vi "MEASURE_hysteresis_multiple_SHG gate_pmt-final - Set voltage.vi"() -> ()   [LabVIEW 2020]
uses:
  <vilib>/DAQmx/read.llb/DAQmx Read.vi
  <vilib>/DAQmx/read.llb/DAQmx Read (Counter U32 1Chan 1Samp).vi
  <vilib>/Analysis/baseanly.llb/Mean (DBL).vi
  <vilib>/DAQmx/create/channels.llb/DAQmx Create Channel (CI-Count Edges).vi
  Program Files/National Instruments/LabVIEW 2019/instr.lib/Keithley 24XX/Public/Data/Read (Multiple Points).vi
  <vilib>/DAQmx/miscellaneous.llb/DAQmx Fill In Error Info.vi
  <vilib>/Utility/file.llb/Write To Spreadsheet File (DBL).vi
  Program Files/National Instruments/LabVIEW 2019/instr.lib/Stanford Research 830/Stanford Research 830.lvlib
  <resource>/objmgr/daqmx.rc
  Program Files/National Instruments/LabVIEW 2019/instr.lib/Keithley 24XX/Keithley 24XX.lvlib
  <vilib>/Analysis/NI_AALBase.lvlib
panel:
  in  "Set voltage (T)":bool=TRUE
  in  "back Vg final Value":dbl=6.0
  in  "Gate sequence":dbl
  out "while loop":dbl
  in  "bottom gate-off set":dbl=-5.0
  in  "0ff set{T}/no off set[F]":bool
  out "XY Graph 4":cluster{dbl[], dbl[]}(graph)
  out "XY Graph 3":cluster{dbl[], dbl[]}(graph)
  out "back gate leaking":dbl=2.469318360898143e-10
  out "top gate voltage":dbl format="%#_13g"
  in  "Compliance  Level (1uA)":dbl=1.9999999995789155e-07
  in  "Source Mode  (0: Voltage)":u16(ring) items=["Voltage", "Current"]
  in  "Serial Configuration":T1={"Baud Rate"=9600, "Parity"=0, "Data Bits"=8, "Stop Bits"=10, "Flow Control"=0} {"Flow Control" items=["None", "XON/XOFF", "RTS/CTS", "XON/XOFF & RTS/CTS", "DTR/DSR", "XON/XOFF & DTR/DSR"]; "Stop Bits" items=["1.0"=10, "1.5"=15, "2.0"=20]; "Data Bits" items=["7"=7, "8"=8]; "Parity" items=["None", "Odd", "Even", "Mark", "Space"]; "Baud Rate" items=["300"=300, "600"=600, "1200"=1200, "2400"=2400, "4800"=4800, "9600"=9600, "19200"=19200]}
  in  "back gate address":refnum<visa-resource-name>="GPIB0::25::INSTR"
  in  "top gate thickness":dbl=10.0
  in  "back gate thickness":dbl=30.0
  in  "pure field (T)/pure doping (F)":bool
  in  "Clear Plot 2":bool
  out "XY Graph 2":cluster{dbl[], dbl[]}(graph)
  in  "accumulation":i32=80
  out "Waveform Chart 3":dbl[](graph)=[376.0, 339.0, 337.0, 347.0, 368.0, 343.0, 313.0, 342.0, 356.0, 353.0, 315.0, 360.0, 375.0, 301.0, 363.0, 324.0, 334.0, 324.0, 318.0, 329.0, 312.0, 341.0, 352.0, 336.0, 351.0, 312.0, 361.0, 339.0, 352.0, 315.0, 360.0, 366.0, 324.0, 343.0, 343.0, 330.0, 340.0, 327.0, 393.0, 330.0, 335.0, 353.0, 360.0, 347.0, 337.0, 336.0, 312.0, 331.0, 326.0, 350.0, 344.0, 328.0, 357.0, 355.0, 356.0, 331.0, 328.0, 340.0, 355.0, 387.0, 371.0, 360.0, 331.0, 339.0, 344.0, 367.0, 343.0, 360.0, 360.0, 370.0, 335.0, 366.0, 323.0, 378.0, 373.0, 358.0]
  out "Numeric":dbl=344.60526315789474
  in  "Counter Channel":tag="/Dev1/PFI0"
  in  "error in":errorcluster
  out "loop run":i32=2
  in  "loop #":i32=2
  in  "Save data or not":bool=TRUE
  in  "path (folder + filename)":string="C:\\Users\\User\\Data\\Jason\\03282019\\ pure_bottom_high_6v_rato3 with light2"
  in  "Clear Plot":bool
  out "LOCKIN Measurement":dbl=0.9110010000000001
  in  "Parameter (1: X)":u16(ring)=1 items=["X"=1, "Y"=2, "R"=3, "Theta"=4, "Channel 1"=5, "Channel 2"=6, "Aux In 1"=7, "Aux In 2"=8, "Aux In 3"=9, "Aux In 4"=10]
  out "back gate voltage":dbl format="%#_13g"
  out "top gate leaking":string="-9.306248E-12\n"
  in  "GATE STEP(mv)":i32=450
  in  "GATE Low Value (default 0)":dbl
  in  "GATE High Value":dbl=18.0
  in  "Function (0: Volts) 2":u16(ring) items=["Volts", "Current", "Resistance"]
  in  "Source Compaliance":dbl=1.000000000000001e-07
  in  "topgate address":refnum<visa-resource-name>="GPIB0::18::INSTR"
  in  "SD stabilization(S) 2":dbl=0.1 format="%#_13g"
  in  "Sine Output Amplitude (1 V) 2":dbl=0.05
  in  "GATE / SD stablization 3":dbl=0.1 format="%#_13g"
  in  "frequency":dbl=50.0 format="%#_13g"
  in  "Input Connection (0: Single-Ended Voltage)":u16(ring) items=["Single-Ended Voltage", "Differential Voltage", "1 MOhm Current Gain", "100 MOhm Current Gain"]
  in  "LOCKIN address":refnum<visa-resource-name>="GPIB0::8::INSTR"
  # "Gate2400(top) Setting"
  # "Lock-in"
  # "Gate2400(back) Setting"
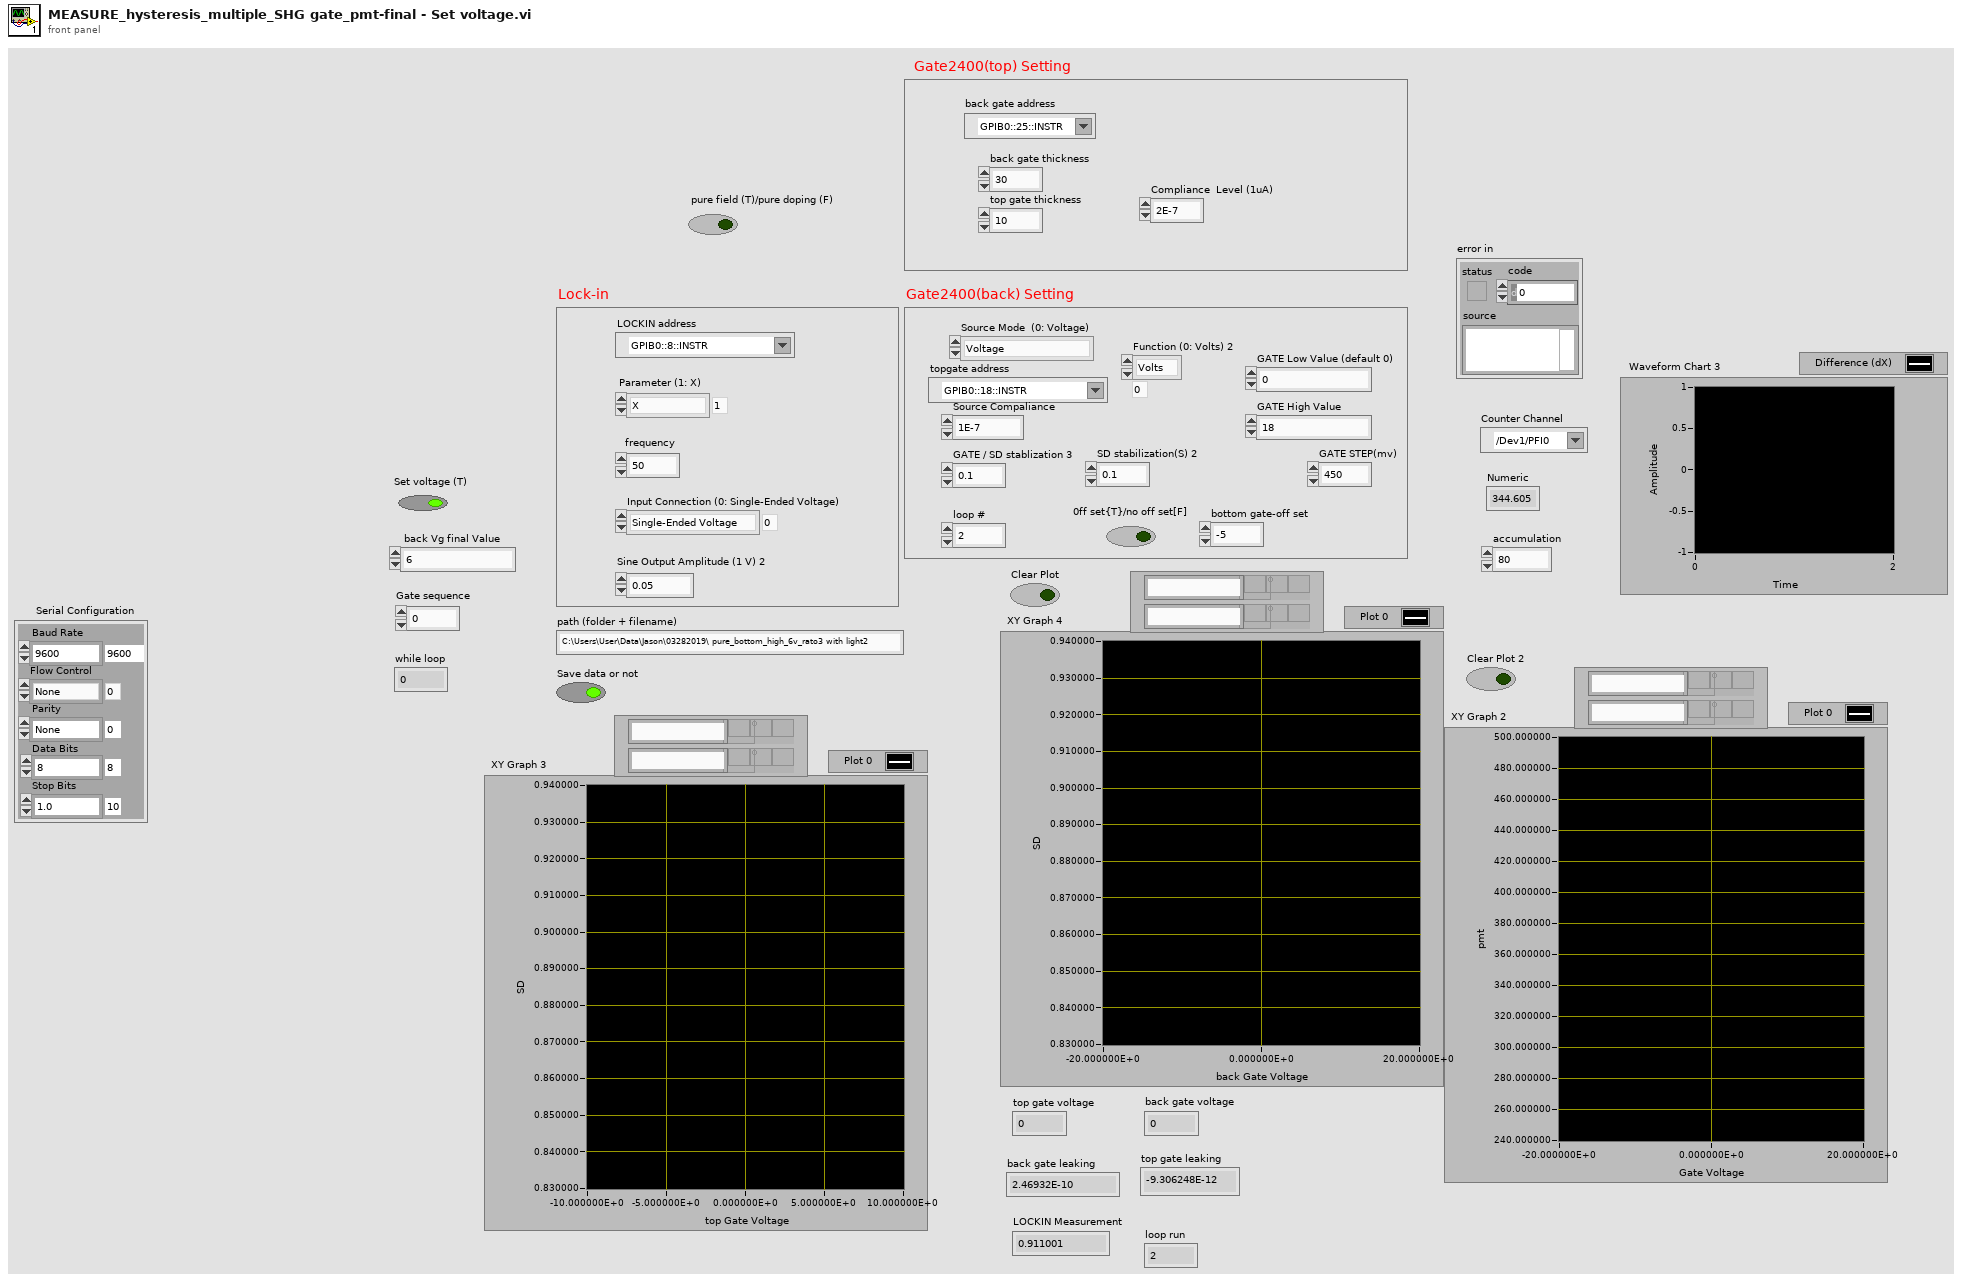
[diagram p1: front panel]
types:
  T1 = cluster{"Baud Rate":u32, "Parity":u16, "Data Bits":u16, "Stop Bits":u16, "Flow Control":u16}
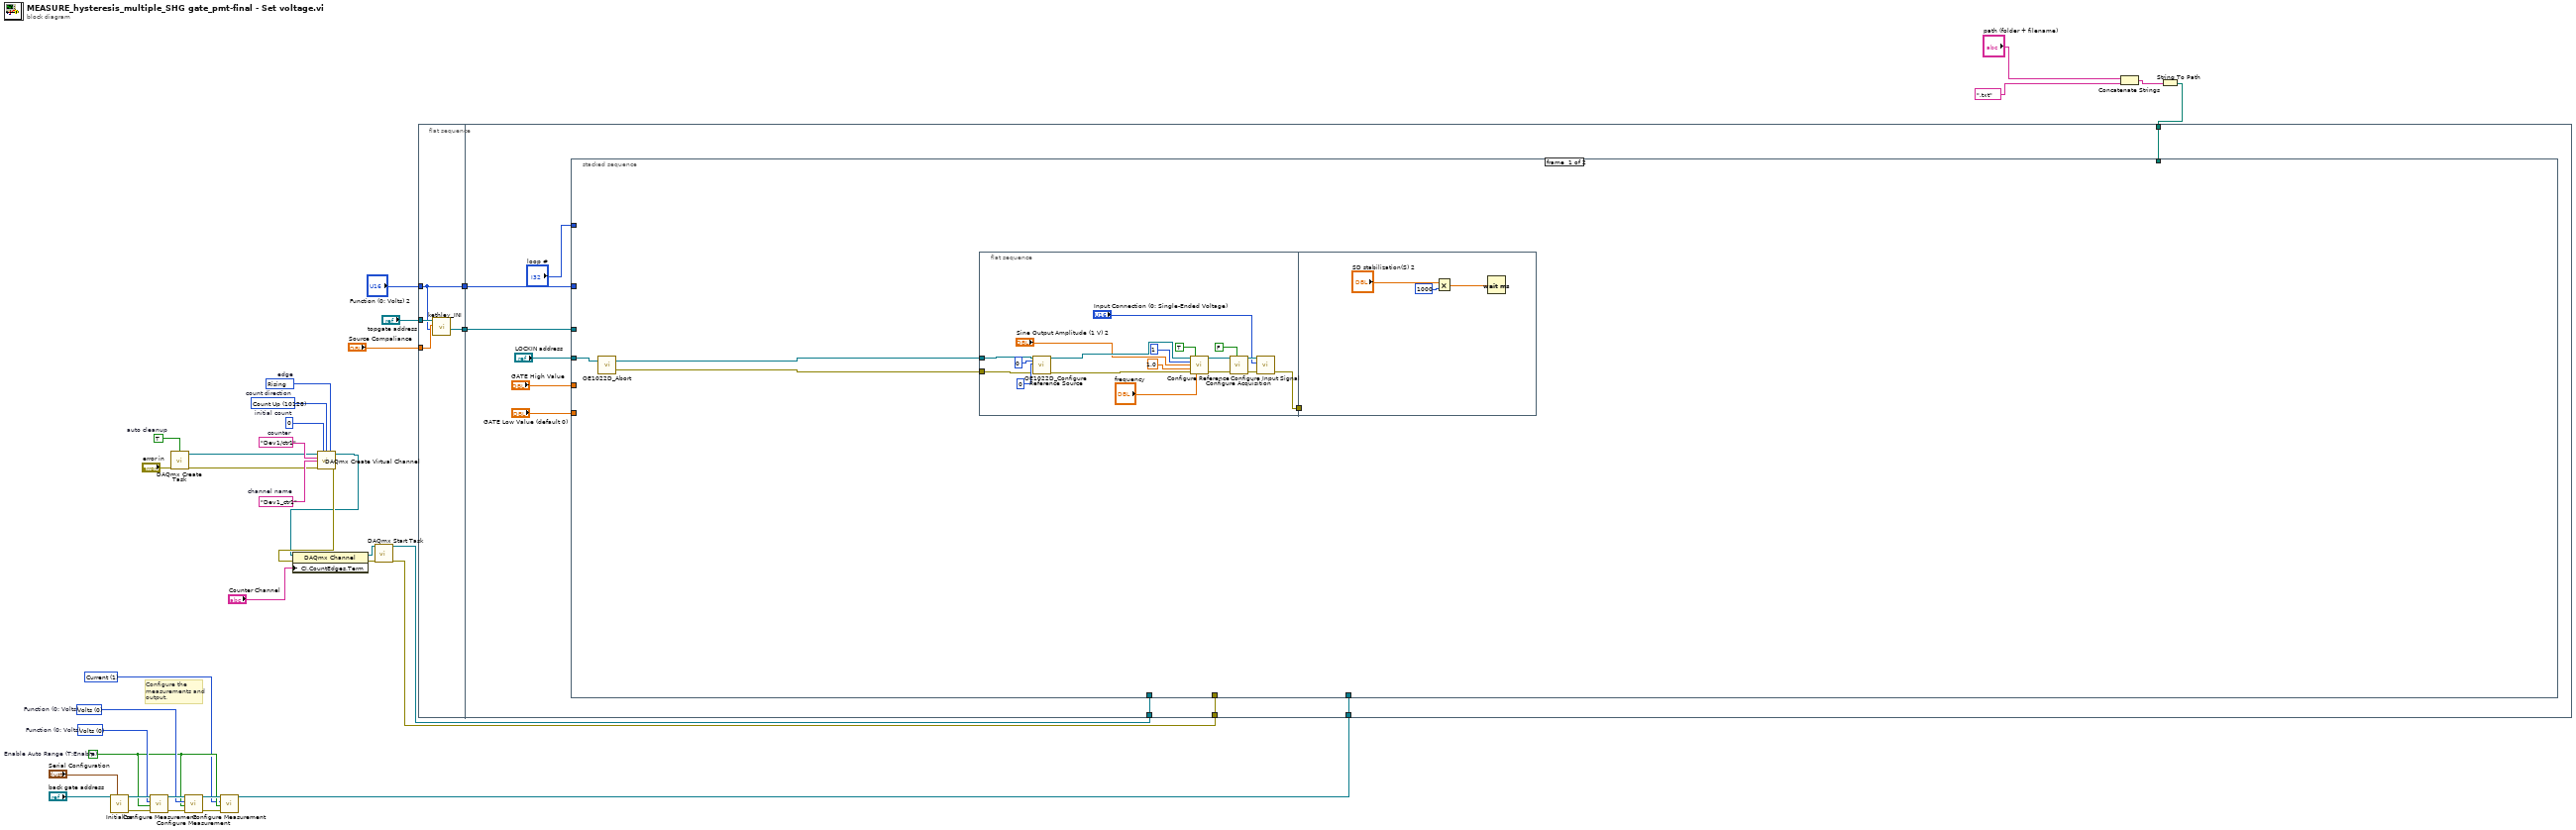
[diagram p0: block diagram]
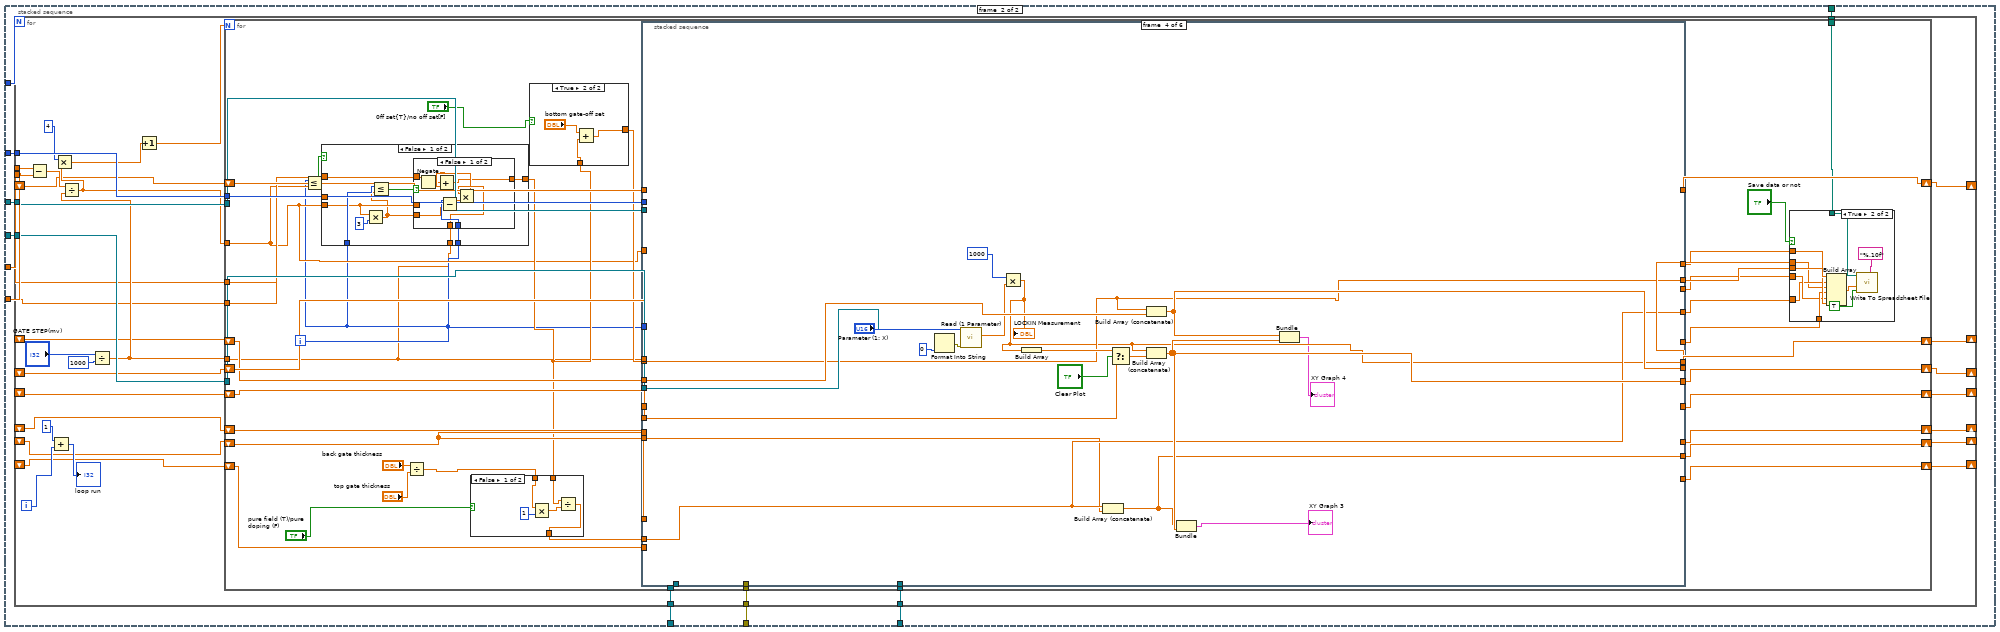
[diagram p2: hidden frame]
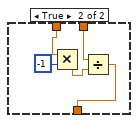
[diagram p4: hidden frame]
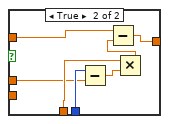
[diagram p6: hidden frame]
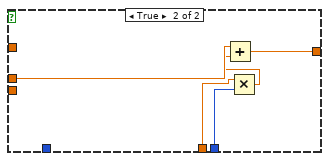
[diagram p7: hidden frame]
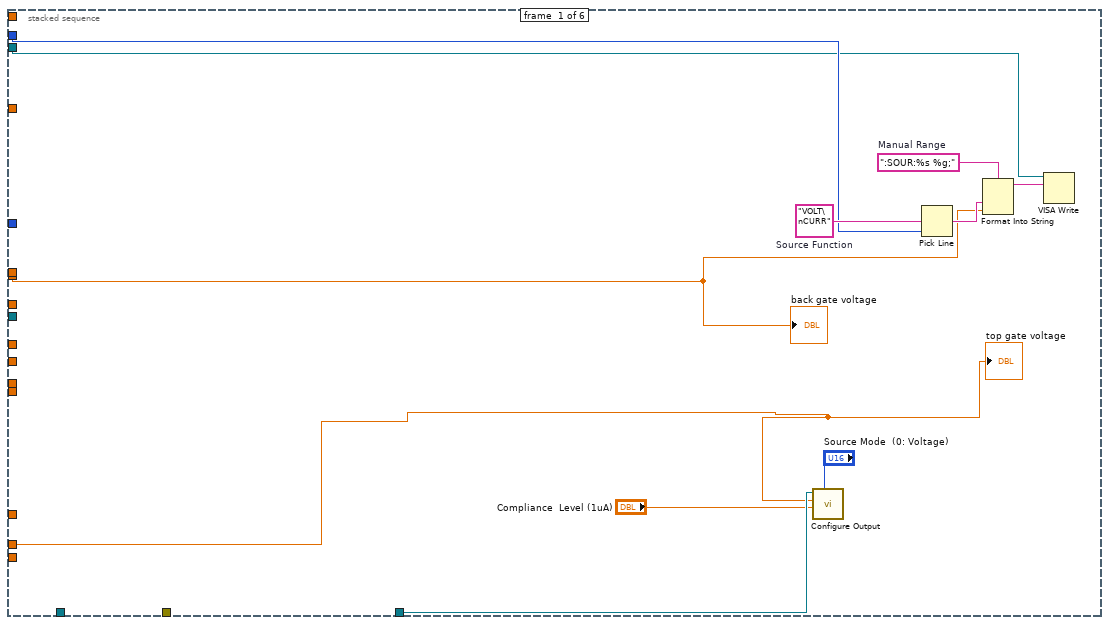
[diagram p8: hidden frame]
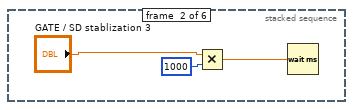
[diagram p9: hidden frame]
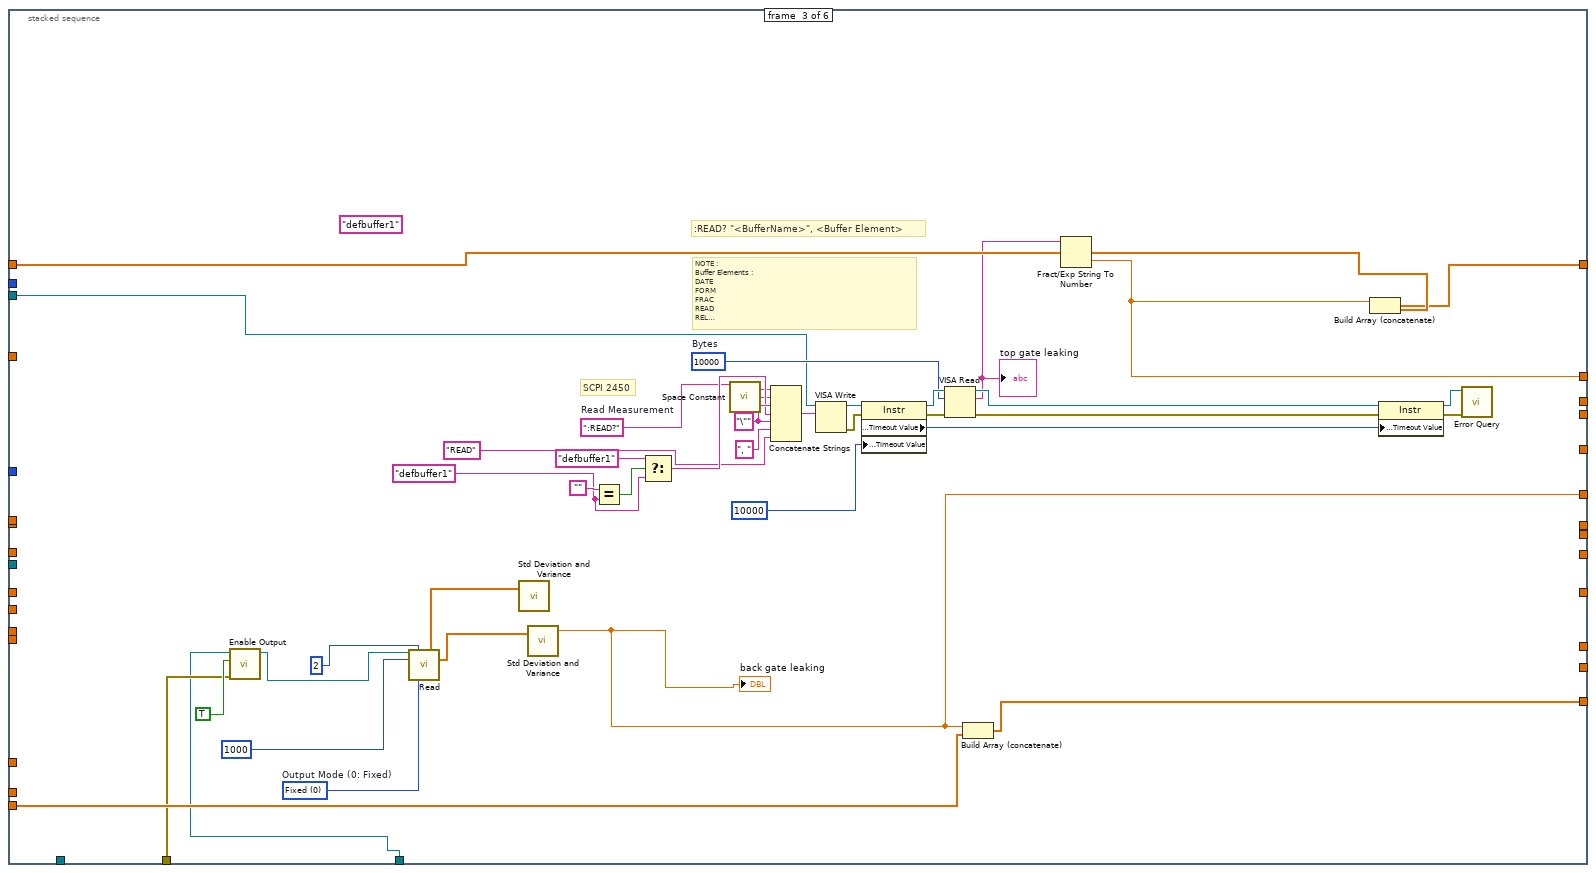
[diagram p10: hidden frame]
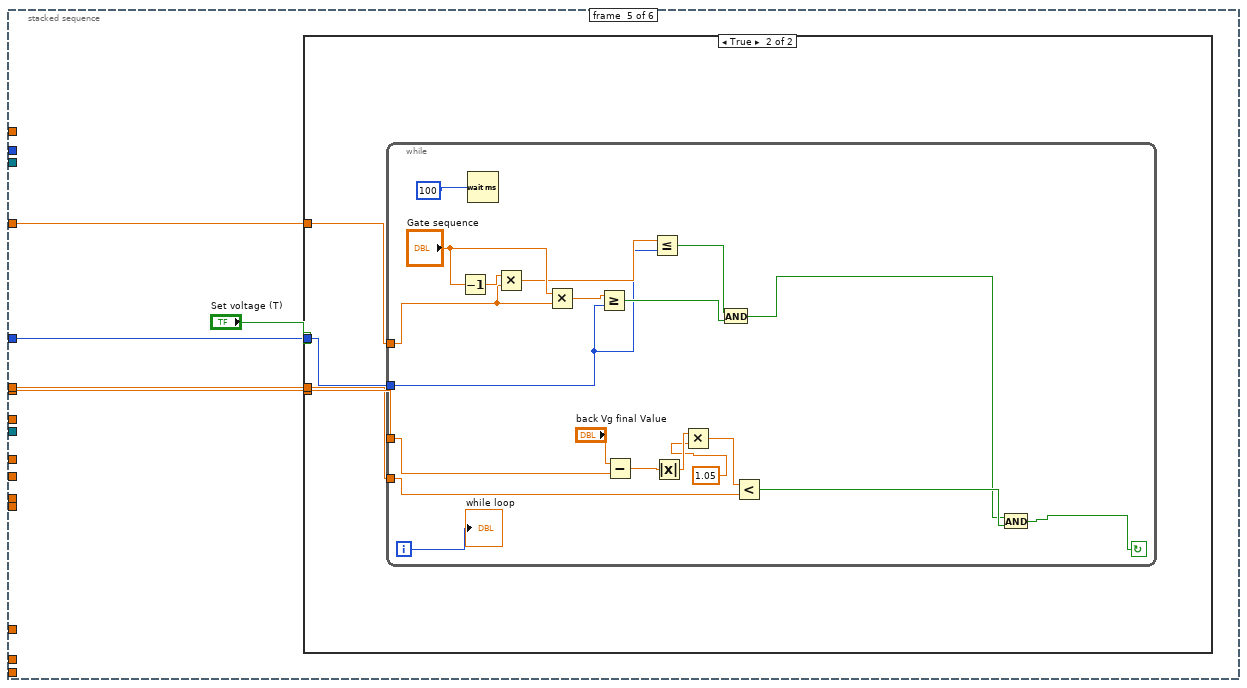
[diagram p11: hidden frame]
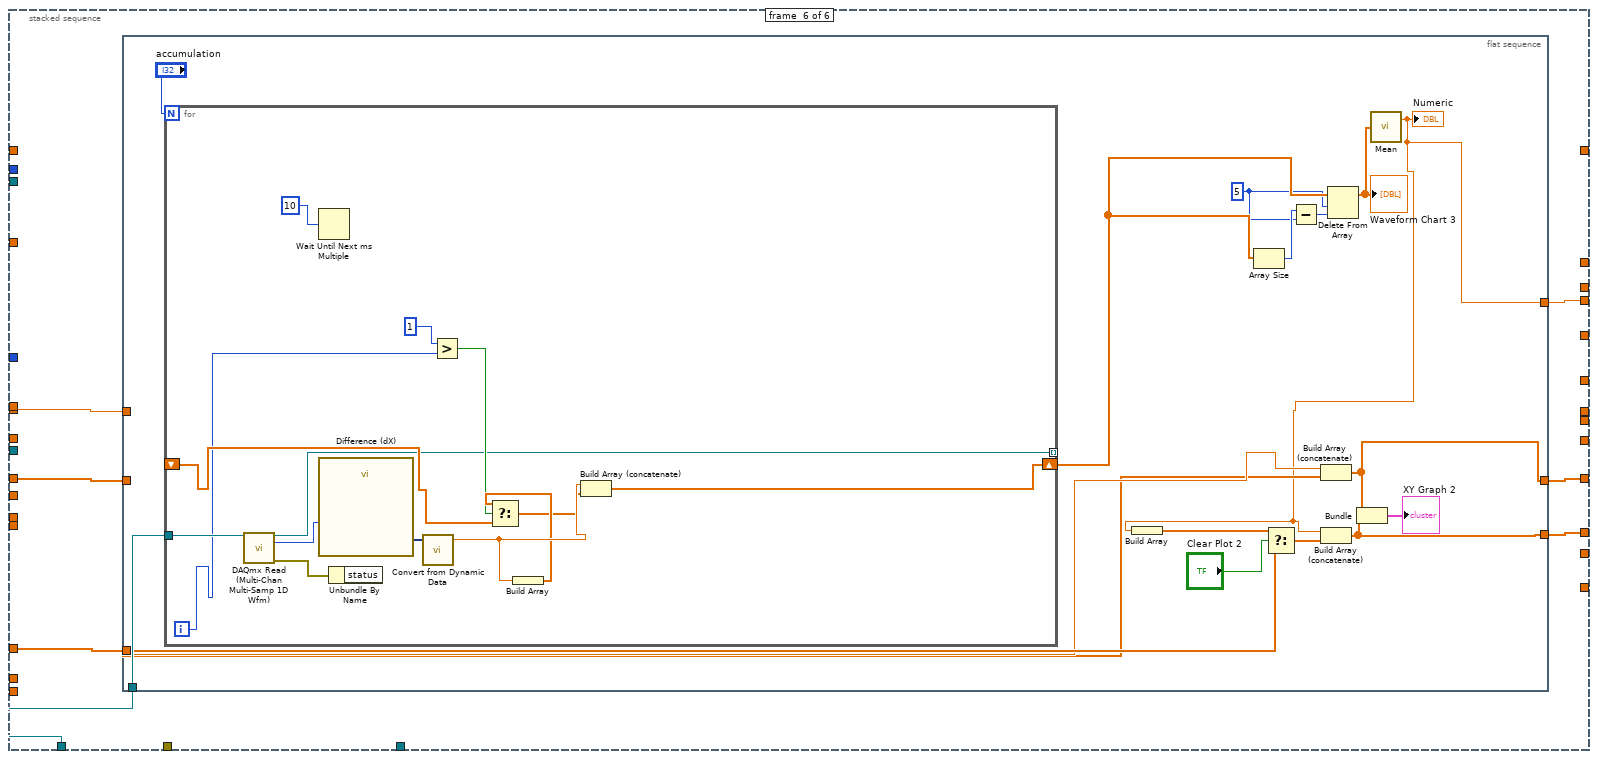
[diagram p13: hidden frame]
diagram:
  w3 = u16 1 items=["Volts", "Current", "Resistance"] ("Function (0: Volts)")
  w4 = TRUE  # Enable Auto Range (T:Enable)
  w7 = u16 0 items=["Volts", "Current", "Resistance"]  # Function (0: Volts)
  w8 = u16 0 items=["Volts", "Current", "Resistance"]  # Function (0: Volts)
  w27 = 10280 items=["Rising"=10280, "Falling"=10171]  # edge
  w26 = 10128 items=["Count Up"=10128, "Count Down"=10124, "Externally Controlled"=10326]  # count direction
  w25 = u32 0  # initial count
  w24 = "Dev1_ctr1"  # channel name
  w23 = "Dev1/ctr1"  # counter
  w21 = TRUE  # auto cleanup
  # "Configure the measurements and output."
  n1 = call "Initialize.vi"("Serial Configuration"="Serial Configuration", "VISA resource name"="back gate address") -> ("error out"=w13:errorcluster, "VISA resource name out"=w14:refnum<visa-resource-name>)  [unwired: 8 in]
  n2 = call "Configure Measurement.vi"("error in (no error)"=w13, "Enable Auto Range (T:Enable)"=w4, "Function (0: Volts)"=w8, "VISA resource name"=w14) -> ("error out"=w12:errorcluster, "VISA resource name out"=w11:refnum<visa-resource-name>)  [unwired: 6 in]
  n3 = call <vilib>:"DAQmx Create Task.vi"("auto cleanup"=w21, "error in"="error in") -> ("task out"=w22:refnum<k21>, "error out"=w20:errorcluster)  [unwired: 12 in]
  n4 = call "Configure Measurement.vi"("error in (no error)"=w12, "Enable Auto Range (T:Enable)"=w4, "Function (0: Volts)"=w7, "VISA resource name"=w11) -> ("error out"=w5:errorcluster, "VISA resource name out"=w6:refnum<visa-resource-name>)  [unwired: 6 in]
  n5 = call "Configure Measurement.vi"("error in (no error)"=w5, "Enable Auto Range (T:Enable)"=w4, "Function (0: Volts)"=w3, "VISA resource name"=w6) -> ("VISA resource name out"=w2:refnum<visa-resource-name>)  [unwired: 6 in, 1 out]
  n6 = call-poly <vilib>:"DAQmx Create Virtual Channel.vi"("task in"=w22, "initial count"=w25, "count direction"=w26, "edge"=w27, "counter"=w23, "name to assign"=w24, "error in"=w20) -> ("task out"=w28:refnum<k21>, "error out"=w29:errorcluster)  [unwired: 7 in]
  n7 = property class="DAQmx Channel"(reference=w28, error in=w29, "CI.CountEdges.Term"="Counter Channel") -> (reference out=w16:refnum<k21>, error out=w17:errorcluster)
  n8 = call <vilib>:"DAQmx Start Task.vi"("task/channels in"=w16, "error in"=w17) -> ("task out"=w15:refnum<k21>, "error out"=w1:errorcluster)  [unwired: 12 in]
  n9 = flat-sequence {
    tunnel: "topgate address" -> [w42]
    tunnel: "Source Compaliance" -> [w41]
    tunnel: "Function (0: Volts) 2" -> [w39]
    tunnel: [w40] -> w35
    tunnel: [w39] -> w34
    tunnel: w35 -> [w51]
    tunnel: w34 -> [w50]
    tunnel: w30 -> [w47]
    tunnel: w15 -> [w45]
    tunnel: w2 -> [w44]
    tunnel: w1 -> [w43]
    frame #0 {
      n10 = call "kethley_INI.vi"("Function (0: Volts) in"=w39, "Source Compaliance"=w41, "VISA Refnum in"=w42) -> ("VISA resource name out"=w40:refnum<visa-resource-name>)  [unwired: 8 in]
    }
    frame #1 {
      n11 = stacked-sequence {
        tunnel: "LOCKIN address" -> [w55 w85]
        tunnel: w51 -> [_ w86]
        tunnel: w50 -> [_ w87]
        tunnel: "GATE High Value" -> [_ w83]
        tunnel: "GATE Low Value (default 0)" -> [_ w84]
        tunnel: w47 -> [_ w82]
        tunnel: "loop #" -> [_ w81]
        tunnel: w45 -> [_ w80]
        tunnel: w44 -> [_ w79]
        tunnel: w43 -> [_ w78]
        frame #0 {
          n12 = call "OE1022D_Abort.vi"("VISA resource name"=w55) -> ("error out"=w53:errorcluster, "VISA resource name out"=w54:refnum<visa-resource-name>)  [unwired: 1 in]
          n13 = flat-sequence {
            tunnel: w54 -> [w74]
            tunnel: [w59] -> w56
            tunnel: w53 -> [w58]
            tunnel: w56 -> [_]
            frame #0 {
              n14 = call "OE1022D_Configure Reference Source.vi"("VISA resource name"=w74, "OE1022D A/B"=0, "Reference Source"=0, "error in (no error)"=w58) -> ("VISA resource name out"=w69:refnum<visa-resource-name>, "error out"=w68:errorcluster)  [unwired: 14 in]
              n15 = call "Configure Reference.vi"("VISA resource name"=w69, "Auto Phase (T: Enabled)"=TRUE, "Reference Source (1: Internal)"=1, "Sine Output Amplitude (1 V)"="Sine Output Amplitude (1 V) 2", "Detection Harmonic Number (1)"=1.0 ("output voltage 2"), "error in (no error)"=w68, "Internal Reference Frequency (1000 Hz)"="frequency") -> ("VISA resource name out"=w66:refnum<visa-resource-name>, "error out"=w61:errorcluster)  [unwired: 7 in]
              n16 = call "Configure Acquisition.vi"("Continuous Storage (T: Enable)"=FALSE, "error in (no error)"=w61, "VISA resource name"=w66) -> ("error out"=w60:errorcluster, "VISA resource name out"=w64:refnum<visa-resource-name>)  [unwired: 7 in]
              n17 = call "Configure Input Signal.vi"("error in (no error)"=w60, "Input Connection (0: Single-Ended Voltage)"="Input Connection (0: Single-Ended Voltage)", "VISA resource name"=w64) -> ("error out"=w59:errorcluster)  [unwired: 7 in, 1 out]
            }
            frame #1 {
              n18 = Multiply(x="SD stabilization(S) 2", y=1000) -> (x*y=w77:dbl)
              n19 = Wait (ms)(milliseconds to wait=w77) -> ()  [unwired: 1 out]
            }
          }
        }
        frame #1 {
          n20 = for {
            N: w81 -> [_]
            tunnel: w87 -> [w121]
            tunnel: w86 -> [w120]
            tunnel: w85 -> [w119]
            tunnel: w84 -> [w113]
            tunnel: w83 -> [w112]
            tunnel: w82 -> [w111]
            shift-right: [w107] -> _
            shift-left: _ -> [w106]
            shift-right: [w105] -> _
            shift-left: _ -> [w103]
            shift-right: [w104] -> _
            shift-left: _ -> [w102]
            tunnel: w80 -> [w98]
            shift-right: [w97] -> _
            shift-left: _ -> [w96]
            shift-right: [w95] -> _
            shift-left: _ -> [w94]
            shift-right: [w93] -> _
            shift-left: _ -> [w92]
            shift-right: [w91] -> _
            shift-left: _ -> [w90]
            tunnel: w79 -> [w89]
            tunnel: w78 -> [w88]
            i -> [w100]
            n21 = Subtract(x=w112, y=w113) -> (x-y=w115:dbl)
            n22 = Add(x=1, y=w100) -> (x+y=→"loop run":i32)
            n23 = Divide(x="GATE STEP(mv)", y=1000) -> (x/y=w114:dbl)
            n24 = Divide(x=w115, y=w114) -> (x/y=w110:dbl)
            n25 = Multiply(x=4, y=w110) -> (x*y=w109:dbl)
            n26 = Increment(x=w109) -> (x+1=w108:dbl)
            n27 = for {
              N: w108 -> [_]
              tunnel: w121 -> [w163]
              tunnel: w120 -> [w162]
              tunnel: w119 -> [w161]
              tunnel: w114 -> [w122]
              shift-right: [w160] -> w107
              shift-left: w106 -> [w159]
              shift-right: [w156] -> w104
              shift-left: w102 -> [w158]
              shift-right: [w155] -> w105
              shift-left: w103 -> [w157]
              tunnel: w110 -> [w124]
              tunnel: w113 -> [w153]
              tunnel: w112 -> [w152]
              tunnel: w111 -> [w148]
              tunnel: w98 -> [w146]
              shift-right: [w145] -> w97
              shift-left: w96 -> [w131]
              shift-right: [w144] -> w95
              shift-left: w94 -> [w143]
              shift-right: [w141] -> w93
              shift-left: w92 -> [w132]
              shift-right: [w140] -> w91
              shift-left: w90 -> [w130]
              tunnel: w89 -> [w138]
              tunnel: w88 -> [w129]
              i -> [w123]
              n28 = Less Or Equal?(x=w123, y=w124) -> (x <= y?=w154:bool)
              n29 = case shown="False" w154 {
                tunnel: w153 -> [_ w216]
                tunnel: w123 -> [w196 w215]
                tunnel: w122 -> [w195 w214]
                tunnel: [w193 w212] -> w126
                tunnel: w152 -> [w194 _]
                tunnel: w124 -> [w189 _]
                tunnel: w123 -> [w192 _]
                frame False {
                  n30 = Multiply(x=w189, y=3) -> (x*y=w188:dbl)
                  n31 = Less Or Equal?(x=w192, y=w188) -> (x <= y?=w190:bool)
                  n32 = case shown="False" w190 {
                    tunnel: w196 -> [w204 w211]
                    tunnel: w195 -> [w202 w209]
                    tunnel: w194 -> [w198 w207]
                    tunnel: [w200 w206] -> w193
                    tunnel: w189 -> [_ w205]
                    tunnel: w188 -> [w197 _]
                    frame False {
                      n33 = Negate(x=w198) -> (-x=w199:dbl)
                      n34 = Subtract(x=w204, y=w197) -> (x-y=w203:dbl)
                      n35 = Multiply(x=w202, y=w203) -> (x*y=w201:dbl)
                      n36 = Add(x=w199, y=w201) -> (x+y=w200:dbl)
                    }
                    frame True {
                      n37 = Subtract(x=w211, y=w205) -> (x-y=w210:dbl)
                      n38 = Multiply(x=w209, y=w210) -> (x*y=w208:dbl)
                      n39 = Subtract(x=w207, y=w208) -> (x-y=w206:dbl)
                    }
                  }
                }
                frame True {
                  n40 = Multiply(x=w214, y=w215) -> (x*y=w213:dbl)
                  n41 = Add(x=w216, y=w213) -> (x+y=w212:dbl)
                }
              }
              n42 = Divide(x="back gate thickness", y="top gate thickness") -> (x/y=w137:dbl)
              n43 = case shown="False" "pure field (T)/pure doping (F)" {
                tunnel: w137 -> [w171 w177]
                tunnel: [w168 w175] -> w133
                tunnel: w126 -> [w169 w174]
                frame False {
                  n44 = Multiply(x=w171, y=1) -> (x*y=w170:dbl)
                  n45 = Divide(x=w169, y=w170) -> (x/y=w168:dbl)
                }
                frame True {
                  n46 = Multiply(x=w177, y=-1) -> (x*y=w173:dbl)
                  n47 = Divide(x=w174, y=w173) -> (x/y=w175:dbl)
                }
              }
              n48 = case shown="True" "0ff set{T}/no off set[F]" {
                tunnel: w126 -> [w164 w167]
                tunnel: [w164 w165] -> w125
                frame False {
                }
                frame True {
                  n49 = Add(x="bottom gate-off set", y=w167) -> (x+y=w165:dbl)
                }
              }
              n50 = stacked-sequence {
                tunnel: w163 -> [w223 _ _ _ _ _]
                tunnel: w162 -> [w222 _ w247 _ _ _]
                tunnel: w161 -> [_ _ _ w281 _ _]
                tunnel: w125 -> [w221 _ _ w280 w291 w321]
                tunnel: [_ _ w245 _ _ _] -> w160
                tunnel: w159 -> [_ _ w246 _ _ _]
                tunnel: w158 -> [_ _ _ w284 _ _]
                tunnel: w157 -> [_ _ _ w282 _ _]
                tunnel: [_ _ _ w277 _ _] -> w156
                tunnel: [_ _ _ w283 _ _] -> w155
                tunnel: [_ _ _ w271 _ _] -> w151
                tunnel: [_ _ _ w280 _ _] -> w150
                tunnel: [_ _ w243 _ _ _] -> w149
                tunnel: w146 -> [_ _ _ _ _ w325]
                tunnel: [_ _ _ _ _ w324] -> w145
                tunnel: w131 -> [_ _ _ _ _ w323]
                tunnel: [_ _ _ _ _ w322] -> w144
                tunnel: w143 -> [_ _ _ _ _ w320]
                tunnel: [_ _ _ _ _ w319] -> w142
                tunnel: [_ _ w237 _ _ _] -> w141
                tunnel: [_ _ _ w276 _ _] -> w140
                tunnel: w130 -> [_ _ _ _ _ _]
                tunnel: [_ _ _ w275 _ _] -> w139
                tunnel: [_ _ w236 _ _ _] -> w128
                tunnel: w138 -> [w219 _ w232 _ _ _]
                tunnel: w133 -> [w217 _ _ w275 _ _]
                tunnel: w132 -> [_ _ w235 _ _ _]
                tunnel: w130 -> [_ _ _ w274 _ _]
                tunnel: w129 -> [_ _ w233 _ _ _]
                tunnel: w124 -> [_ _ _ _ w293 _]
                tunnel: w123 -> [_ _ _ _ w292 _]
                tunnel: w122 -> [_ _ _ _ w290 _]
                frame #0 {
                  w225 = "VOLT\nCURR"  # Source Function
                  w226 = ":SOUR:%s %g;"  # Manual Range
                  n51 = call "Configure Output.vi"("Source Mode  (0: Voltage)"="Source Mode  (0: Voltage)", "Compliance  Level (0.1)"="Compliance  Level (1uA)", "Output Level (0)"=w217, "VISA resource name"=w219) -> ()  [unwired: 6 in, 2 out]
                  n52 = Pick Line(multi-line string=w225, line index=w223) -> (output string=w224:string)  [unwired: 1 out]
                  n53 = Format Into String(format string=w226, w224, w221) -> (resulting string=w227:string)  [unwired: 2 in, 1 out]
                  n54 = VISA Write(VISA resource name=w222, write buffer=w227) -> ()  [unwired: 1 in, 3 out]
                  "back gate voltage" <- w221
                  "top gate voltage" <- w217
                }
                frame #1 {
                  n55 = Multiply(x="GATE / SD stablization 3", y=1000) -> (x*y=w230:dbl)
                  n56 = Wait (ms)(milliseconds to wait=w230) -> ()  [unwired: 1 out]
                }
                frame #2 {
                  w240 = u16 0 items=["Fixed", "Sweep", "List"]  # Output Mode (0: Fixed)
                  w258 = "defbuffer1" ("Buffer Name (defbuffer1) 2")
                  (unwired) "defbuffer1" ("t")
                  w256 = "\""
                  w253 = ":READ?"  # Read Measurement
                  w262 = u32 10000  # Bytes
                  # "NOTE :\nBuffer Elements :\nDATE\nFORM\nFRAC\nREAD\nREL\nSEC\nSOUR\nSOURFORM\nSOURSTAT\nSOURUNIT\nSTAT\nTIME\nTsT\nUNIT"
                  # ":READ? \"<BufferName>\", <Buffer Element>"
                  # "SCPI 2450"
                  n57 = call "Enable Output.vi"("error in (no error)"=w233, "Enable Output (T: Enable)"=TRUE, "VISA resource name"=w232) -> ("VISA resource name out"=w231:refnum<visa-resource-name>)  [unwired: 7 in, 1 out]
                  n58 = call-poly "Read.vi"("VISA resource name"=w231, "Sample Count (1)"=u32 2 ("Number of Samples"), "Timeout (10000 ms)"=1000, "Output Mode (0: Fixed)"=w240) -> ("Voltage"=w238:sgl[], "Current"=w239:sgl[])  [unwired: 5 in, 5 out]
                  n59 = call <vilib>:"Std Deviation and Variance.vi"("X"=w238) -> ()  [unwired: 1 in, 3 out]
                  n60 = call <vilib>:"Std Deviation and Variance.vi"("X"=w239) -> ("mean"=w236:dbl)  [unwired: 1 in, 2 out]
                  "back gate leaking" <- w236
                  n61 = Equal?(x="", y=w258) -> (x = y?=w259:bool)
                  n62 = Select(t="defbuffer1", s=w259, f=w258) -> (s? t:f=w255:string)
                  n63 = call <vilib>:"Space Constant.vi"() -> ("String"=w254:string)
                  n64 = Concatenate Strings(w253, w254, w256, w255, w256, ", " ("string"), "READ" ("Buffer Elements 2")) -> (w269:string)
                  n65 = VISA Write(VISA resource name=w247, write buffer=w269) -> (VISA resource name out=w261:refnum<visa-resource-name>, error out=w268:errorcluster)  [unwired: 1 in, 1 out]
                  n66 = property class="Instr"(reference=w261, error in=w268, "General Settings:Timeout Value"=10000 ("Timeout (10000 ms) 2")) -> (reference out=w267:refnum<visa-resource-name>, error out=w266:errorcluster, "General Settings:Timeout Value"=w263:u32)
                  n67 = VISA Read(VISA resource name=w267, byte count=w262, error in (no error)=w266) -> (VISA resource name out=w265:refnum<visa-resource-name>, read buffer=w244:string, error out=w264:errorcluster)  [unwired: 1 out]
                  "top gate leaking" <- w244
                  n68 = Build Array (concatenate)(w236, w235) -> (w237:dbl[])
                  n69 = Fract/Exp String To Number(string=w244) -> (number=w243:dbl)  [unwired: 3 in, 1 out]
                  n70 = Build Array (concatenate)(w243, w246) -> (w245:dbl[])
                  n71 = property class="Instr"(reference=w265, error in=w264, "General Settings:Timeout Value"=w263) -> (reference out=w251:refnum<visa-resource-name>, error out=w250:errorcluster)
                  n72 = call "Error Query.vi"("error in (no error)"=w250, "VISA resource name"=w251) -> ()  [unwired: 6 in, 4 out]
                }
                frame #3 {
                  n73 = Format Into String(0) -> (error out=w289:errorcluster)  [unwired: 3 in, 1 out]
                  n74 = call "Read (1 Parameter).vi"("error in (no error)"=w289, "Parameter (1: X)"="Parameter (1: X)", "VISA resource name"=w281) -> ("Measurement"=w272:dbl)  [unwired: 6 in, 2 out]
                  n75 = Multiply(x=1000, y=w272) -> (x*y=w271:dbl)
                  "LOCKIN Measurement" <- w271
                  n76 = Build Array(w271) -> (w287:dbl[])
                  n77 = Build Array (concatenate)(w275, w274) -> (w276:dbl[])
                  n78 = Select(t=w287, s="Clear Plot", f=w284) -> (s? t:f=w279:dbl[])
                  n79 = Build Array (concatenate)(w280, w282) -> (w283:dbl[])
                  n80 = Build Array (concatenate)(w271, w279) -> (w277:dbl[])
                  n81 = Bundle(w276, w277) -> (→"XY Graph 3":cluster{dbl[], dbl[]})  [unwired: 1 in]
                  n82 = Bundle(w283, w277) -> (→"XY Graph 4":cluster{dbl[], dbl[]})  [unwired: 1 in]
                }
                frame #4 {
                  n83 = case shown="True" "Set voltage (T)" {
                    tunnel: w293 -> [_ w298]
                    tunnel: w292 -> [_ w297]
                    tunnel: w291 -> [_ w296]
                    tunnel: w290 -> [_ w295]
                    frame False {
                    }
                    frame True {
                      n84 = while {
                        tunnel: w297 -> [w304]
                        tunnel: w298 -> [w308]
                        tunnel: w295 -> [w313]
                        tunnel: w296 -> [w311]
                        i -> [w318]
                        stop <- w316 continue-if-true
                        n85 = Decrement(x="Gate sequence") -> (x-1=w309:dbl)
                        n86 = Wait (ms)(milliseconds to wait=100) -> ()  [unwired: 1 out]
                        n87 = Multiply(x=w309, y=w308) -> (x*y=w305:dbl)
                        n88 = Multiply(x="Gate sequence", y=w308) -> (x*y=w307:dbl)
                        n89 = Greater Or Equal?(x=w307, y=w304) -> (x >= y?=w306:bool)
                        n90 = Subtract(x="back Vg final Value", y=w311) -> (x-y=w314:dbl)
                        n91 = Less Or Equal?(x=w305, y=w304) -> (x <= y?=w303:bool)
                        n92 = Absolute Value(x=w314) -> (abs(x)=w301:dbl)
                        n93 = Multiply(x=w301, y=1.05) -> (x*y=w300:dbl)
                        n94 = And(x=w303, y=w306) -> (x .and. y?=w302:bool)
                        n95 = Less?(x=w300, y=w313) -> (x < y?=w312:bool)
                        n96 = And(x=w302, y=w312) -> (x .and. y?=w316:bool)
                        "while loop" <- w318
                      }
                    }
                  }
                }
                frame #5 {
                  n97 = flat-sequence {
                    tunnel: w325 -> [w337]
                    tunnel: [w330] -> w324
                    tunnel: w323 -> [w331]
                    tunnel: [w329] -> w322
                    tunnel: w321 -> [w328]
                    tunnel: w320 -> [w327]
                    tunnel: [w326] -> w319
                    frame #0 {
                      w339 = 5
                      n98 = for {
                        N: "accumulation" -> [_]
                        tunnel: w337 -> [w347]
                        shift-right: [w346] -> w341
                        shift-left: _ -> [w345]
                        tunnel: [w343] -> _ mode=indexing
                        i -> [w344]
                        n99 = call-poly "DAQmx Read (Multi-Chan Multi-Samp 1D Wfm).vi"("task/channels in"=w347) -> ("task out"=w343:refnum<k21>, "data"=w353:u32, "error out"=w354:errorcluster)  [unwired: 12 in]
                        n100 = Wait Until Next ms Multiple(millisecond multiple=10) -> ()  [unwired: 1 out]
                        n101 = call "Difference (dX)"("Signals"=w353) -> ("Result"=w356:dynamicdata)  [unwired: 5 in, 1 out]
                        n102 = Unbundle By Name(w354) -> ()  [unwired: 1 out]
                        n103 = call "Convert from Dynamic Data"("Dynamic Data Type"=w356) -> ("Scalar"=w352:dbl)  [unwired: 3 in]
                        n104 = Greater?(x=1, y=w344) -> (0:w348:bool)
                        n105 = Build Array(w352) -> (w351:dbl[])
                        n106 = Select(t=w351, s=w348, f=w345) -> (s? t:f=w350:dbl[])
                        n107 = Build Array (concatenate)(w352, w350) -> (w346:dbl[])
                      }
                      n108 = Array Size(array=w341) -> (size(s)=w340:i32)
                      n109 = Subtract(x=w340, y=w339) -> (x-y=w338:i32)
                      n110 = Build Array (concatenate)(w328, w327) -> (w329:dbl[])
                      n111 = Delete From Array(array=w341, length=w339, index=w338) -> (array with subset deleted=w336:dbl[])  [unwired: 1 out]
                      "Waveform Chart 3" <- w336
                      n112 = call-poly <vilib>:"Mean.vi"("X"=w336) -> ("mean"=w326:dbl)  [unwired: 1 out]
                      "Numeric" <- w326
                      n113 = Build Array(w326) -> (w334:dbl[])
                      n114 = Select(t=w334, s="Clear Plot 2", f=w331) -> (s? t:f=w335:dbl[])
                      n115 = Build Array (concatenate)(w326, w335) -> (w330:dbl[])
                      n116 = Bundle(w329, w330) -> (→"XY Graph 2":cluster{dbl[], dbl[]})  [unwired: 1 in]
                    }
                  }
                }
              }
              n117 = case shown="True" "Save data or not" {
                tunnel: w151 -> [_ w178]
                tunnel: w150 -> [_ w187]
                tunnel: w149 -> [_ w186]
                tunnel: w148 -> [_ w184]
                tunnel: w142 -> [_ w180]
                tunnel: w139 -> [_ w179]
                tunnel: w128 -> [_ w181]
                frame False {
                }
                frame True {
                  n118 = Build Array(w187, w179, w178, w181, w180, w186) -> (w185:dbl[])
                  n119 = call-poly <vilib>:"Write To Spreadsheet File.vi"("format (%.3f)"="%.10f", "append to file? (new file:F)"=TRUE, "1D data"=w185, "file path (dialog if empty)"=w184) -> ()  [unwired: 4 in, 1 out]
                }
              }
            }
          }
        }
      }
    }
  }
  n120 = Concatenate Strings("path (folder + filename)", ".txt") -> (w31:string)
  n121 = String To Path(string=w31) -> (path=w30:path)
